vi "ReadString.vi"(8 "error in (no error)":errorcluster, 10 "Timeout":u32, 11 "StringReader in":refnum<class "StringReader.lvclass">) -> (0 "error out":errorcluster, 2 "String":string, 3 "StringReader out":refnum<class "StringReader.lvclass">)   [LabVIEW 2013, in "StringReader.lvclass"]
doc: "Read a string from the remote destination"
uses:
  StringReader.lvclass
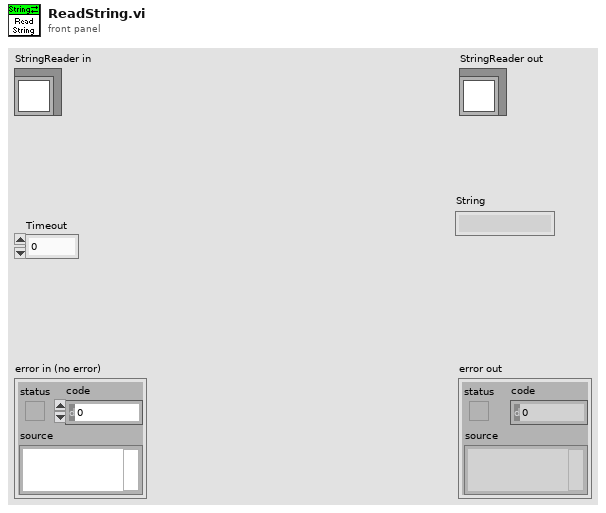
[diagram p1: front panel]
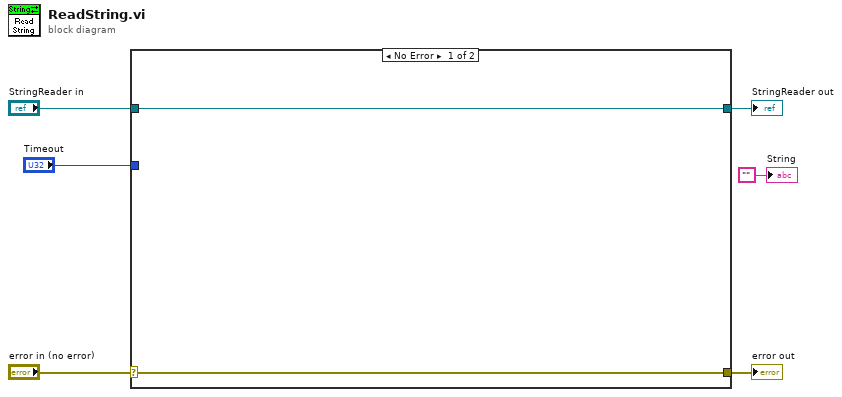
[diagram p0: block diagram]
diagram:
  n1 = case shown="No Error" "error in (no error)" {
    selector: "error in (no error)" -> [w7 w10]
    tunnel: [w7 w10] -> w5
    tunnel: [w8 w9] -> w3
    tunnel: "StringReader in" -> [w8 w9]
    tunnel: "Timeout" -> [_ _]
    frame No Error {
    }
    frame Error {
    }
  }
  "error out" <- w5
  "StringReader out" <- w3
  "String" <- ""
